vi "Describe First Encoded Error.vi"(11 "error in":errorcluster) -> (1 "encoded":bool, 3 "tokens":cluster{"token type":T1, T2}[](array[cluster]))   [LabVIEW 2020, in "Multi Error Cluster.lvlib"]
doc: "Tokenize the first element of a multi-error or encoded error."
uses:
  <vilib>/MultiError/TokenizeJSON/Multi Error Cluster.lvlib
  <vilib>/MultiError/TokenizeJSON/JSON Token Values.ctl
  <vilib>/MultiError/Errors Cluster Multiple Errors/JSON Token Descriptor.ctl
  <vilib>/MultiError/TokenizeJSON/JSON Raw Token Values.ctl
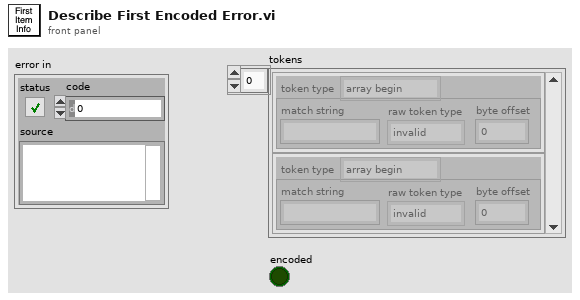
[diagram p1: front panel]
types:
  T1 = typedef "Multi Error Cluster.lvlib/JSON Token Values.ctl" = enum32{"array begin", "array end", "object begin", "object end", "value", "invalid", "name"}
  T2 = typedef "Multi Error Cluster.lvlib/JSON Token Descriptor.ctl" = cluster{"match string":string, "raw token type":T3, "byte offset ":i32}
  T3 = typedef "Multi Error Cluster.lvlib/JSON Raw Token Values.ctl" = enum32{"{", "}", "[", "]", ",", ":", "\"", "number", "string", "true", "false", "null", "invalid"}
  T4 = typedef "Multi Error Cluster.lvlib/JSON Object Descriptor.ctl" = cluster{"begin info":T2, "end info":T2, "begin Index":i32, "end Index":i32}
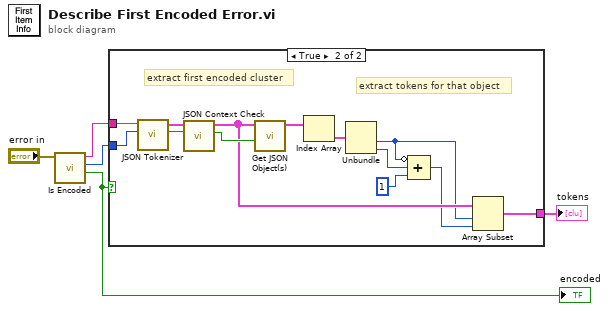
[diagram p0: block diagram]
diagram:
  n1 = call <vilib>:"Is Encoded.vi"("error in (no error)"="error in") -> ("Is Encoded"=w5:bool, "offset past"=w3:i32, "source"=w4:string)  [unwired: 8 in]
  "encoded" <- w5
  n2 = case shown="True" w5 {
    tunnel: w4 -> [_ w14]
    tunnel: w3 -> [_ w16]
    tunnel: [_ w6] -> w2
    frame False {
    }
    frame True {
      # "extract tokens for that object"
      # "extract first encoded cluster"
      n3 = call <vilib>:"JSON Tokenizer.vi"("string offset"=w16, "JSON String"=w14) -> ("Invalid"=w17:bool, "Array"=w18:T2[])  [unwired: 8 in]
      n4 = call <vilib>:"JSON Context Check.vi"("Invalid in"=w17, "Parse Tokens in"=w18) -> ("Invalid out"=w15:bool, "tokens"=w9:cluster{"token type":T1, T2}[])  [unwired: 8 in]
      n5 = call <vilib>:"Get JSON Object(s).vi"("invalid in"=w15, "tokens"=w9) -> ("array of JSON objects"=w13:T4[])  [unwired: 9 in]
      n6 = Index Array(array=w13) -> (element=w12:T4)  [unwired: 1 in]
      n7 = Unbundle(w12) -> ("begin Index"=w7:i32, "end Index"=w10:i32)  [unwired: 2 out]
      n8 = Compound Arithmetic op=ADD(invert w7, w10, 1) -> (w8:i32)
      n9 = Array Subset(array=w9, index=w7, length=w8) -> (w6:cluster{"token type":T1, T2}[])
    }
  }
  "tokens" <- w2
